vi "myRIO_BRig_Host_parse_dataTrial__v4.vi"(0 "input_idxReward":i32, 1 "input_arrayReward":i32[][](array[numeric]), 2 "input_idxWrong":i32, 3 "input_arrayWrong":i32[][](array[numeric]), 4 "input_idxTimeout":i32, 5 "input_arrayTimeout":i32[][](array[numeric]), 6 "input_arrayUnknown":i32[][](array[numeric]), 8 "input_idxUnknown":i32, 12 "input_minTrial":i32) -> (14 "output_plotData":cluster{i32[], i32[]}[](array[cluster]))   [LabVIEW 2014]
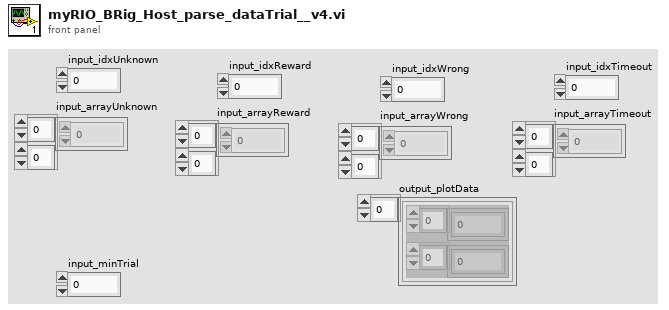
[diagram p1: front panel]
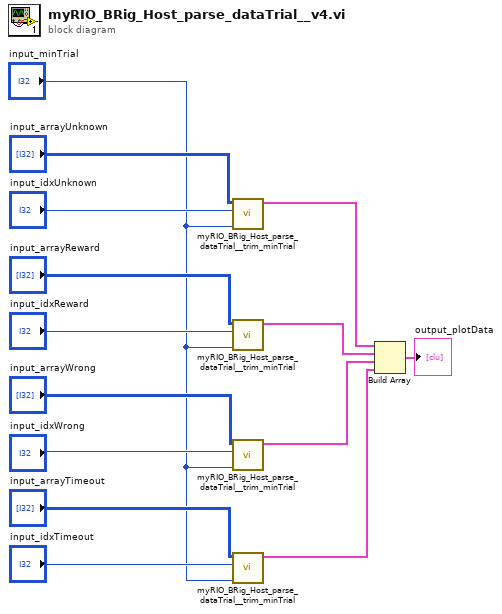
[diagram p0: block diagram]
diagram:
  n1 = call "myRIO_BRig_Host_parse_dataTrial__trim_minTrial.vi"("input_minTrial"="input_minTrial", "input_idx"="input_idxUnknown", "input_array"="input_arrayUnknown") -> ("output_cluster"=w12:cluster{i32[], i32[]})  [unwired: 8 in]
  n2 = call "myRIO_BRig_Host_parse_dataTrial__trim_minTrial.vi"("input_minTrial"="input_minTrial", "input_idx"="input_idxReward", "input_array"="input_arrayReward") -> ("output_cluster"=w8:cluster{i32[], i32[]})  [unwired: 8 in]
  n3 = call "myRIO_BRig_Host_parse_dataTrial__trim_minTrial.vi"("input_minTrial"="input_minTrial", "input_idx"="input_idxWrong", "input_array"="input_arrayWrong") -> ("output_cluster"=w5:cluster{i32[], i32[]})  [unwired: 8 in]
  n4 = call "myRIO_BRig_Host_parse_dataTrial__trim_minTrial.vi"("input_minTrial"="input_minTrial", "input_idx"="input_idxTimeout", "input_array"="input_arrayTimeout") -> ("output_cluster"=w3:cluster{i32[], i32[]})  [unwired: 8 in]
  n5 = Build Array(w12, w8, w5, w3) -> (→"output_plotData":cluster{i32[], i32[]}[])
